vi "pl1000Ready.vi"(8 "error in (no error)":errorcluster, 11 "pl1000 handle":i16) -> (0 "error out":errorcluster, 2 "ready":bool, 3 "pl1000 handle out":i16)   [LabVIEW 2016, in "pl1000.lvlib"]
doc: "This function indicates when pl1000Run has captured the requested number of samples."
uses:
  pl1000.lvlib
  pl1000.dll
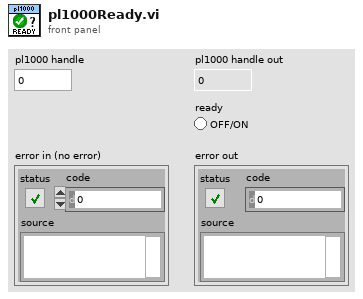
[diagram p1: front panel]
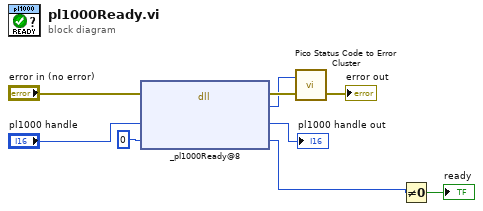
[diagram p0: block diagram]
diagram:
  n1 = dll-call lib="pl1000.dll" fn="_pl1000Ready@8"(error in="error in (no error)", "handle"="pl1000 handle", "ready"=u16 0 ("maxValue")) -> (error out=w7:errorcluster, "status"=w6:u32, "handle"=→"pl1000 handle out":i16, "ready"=w2:i16)  [unwired: 2 in, 1 out]
  n2 = call "Pico Status Code to Error Cluster.vi"("error in"=w7, "PICO_STATUS"=w6) -> ("error out"=→"error out":errorcluster)  [unwired: 1 in]
  n3 = Not Equal To 0?(x=w2) -> (x != 0?=→"ready":bool)
